vi "Qudi_HiM_QPD_PID.vi"(3 "N Z positions":i32) -> ()   [LabVIEW 2015]
uses:
  <vilib>/rvi/Analysis/control/PID/Typedef/niFpgaPID_PIGains.ctl
  <vilib>/Platform/TimedLoop/XDataNode/timing_clust.ctl
  <vilib>/Platform/TimedLoop/XDataNode/nitl_modes.ctl
  <vilib>/Platform/TimedLoop/XDataNode/wakeup.ctl
  <vilib>/rvi/FXPMathLib/basic elements/FxpIntAccumulator/subVIs/nifxpmath_IntAccumulator_SimConfig.ctl
  <vilib>/rvi/Emulation/niFpgaGetClockAttributes.vi
  <vilib>/rvi/Emulation/niFpgaSctlEmulationGetInTimedLoop.vi
  <vilib>/rvi/Emulation/niFpgaEmulationReportErrorSimple.vi
  <vilib>/rvi/eio/common/nirviEmuTemplateMethod_errors.vi
  <vilib>/rvi/Emulation/niFpgaProcessEmulError.vi
  <vilib>/rvi/Analysis/common/codeGenErrors/XNode/niFpgaXNodeCodeGenErrorHandle.vi
  <vilib>/rvi/Emulation/niFpgaCriticalErrorInLSC.vi
  <vilib>/rvi/FXPMathLib/basic elements/FxpIntAccumulator/simVIs/DllFxpIntAccumulator_sub.vi
  <vilib>/rvi/Analysis/control/PID/SubVIs/niFpgaPID_PIWrapper.vi
  <vilib>/eio/EIONode/EIONode.xnode
  <vilib>/rvi/Analysis/measure/dc-rms/XNode/niFpgaDC-RMS.xnode
  <vilib>/Platform/TimedLoop/XDataNode/XDataNode.xnode
  <vilib>/rvi/FXPMathLib/basic elements/FxpIntAccumulator/XNode/nifxpmath_IntAccumulator.xnode
  <vilib>/Platform/TimedLoop/XDataNode/XDNodeRunTimeDep.lvlib
panel:
  in  "integration_time_us":u32=100 caption="Count(uSec)"
  in  "stop":bool
  out "duration_ms":u32
  out "X":i16
  out "Y":i16
  out "Sum":i16
  out "counter":u32
  out "output":i16
  in  "reset":bool
  in  "reset_counter":bool
  in  "autofocus":bool
  in  "setpoint":i16
  in  "P":i16
  in  "I":i16
  in  "ref_axis":bool
  out "n cycles":i32
  out "DIo2":i32
  out "DIo3":i32
  out "DIo1":i32
  out "Images acquired":i32
  in  "Laser lines":i32[](array[numeric])=[0, 0, 0, 0, 0]
  in  "Laser power":i16[](array[numeric])=[0, 0, 0, 0, 0]
  in  "N laser lines":i32
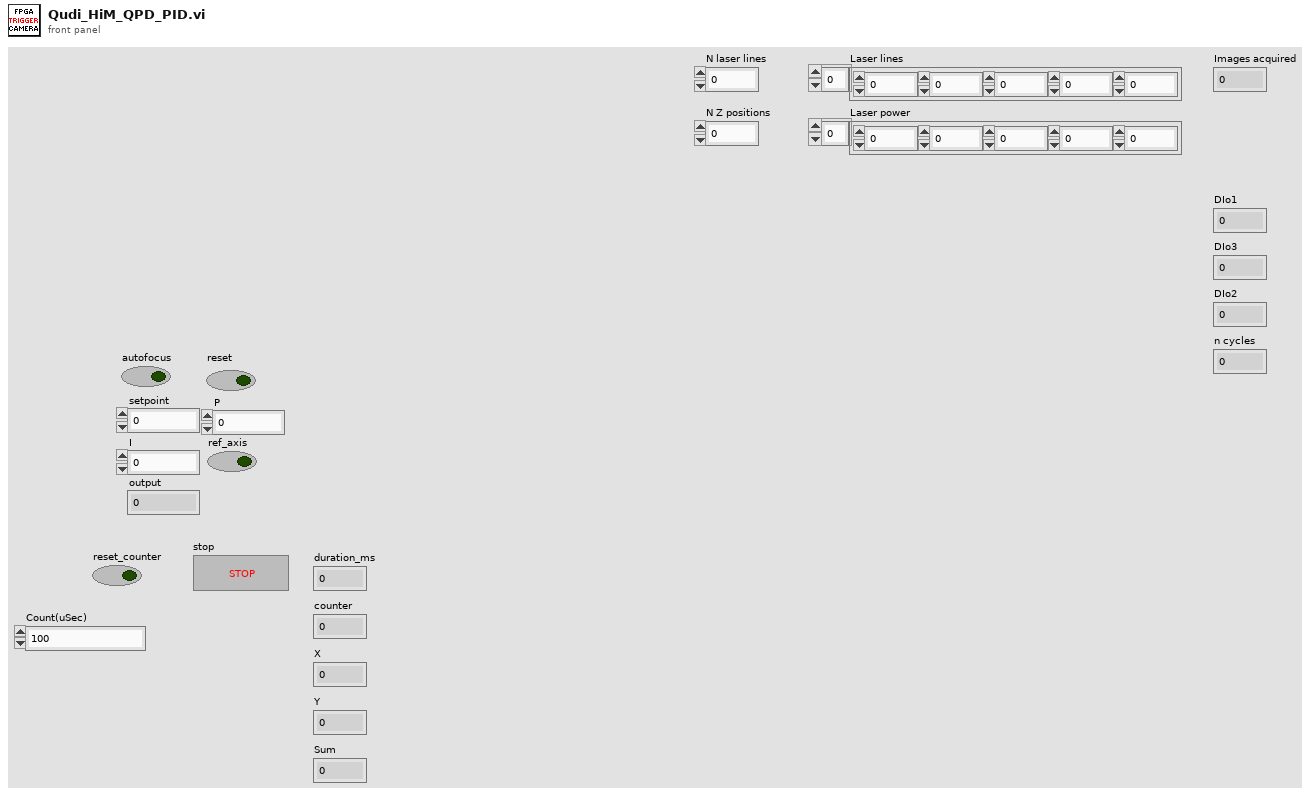
[diagram p1: front panel]
types:
  T1 = typedef "niFpgaPID_PIGains.ctl" = cluster{"proportional gain":sgl, "integral gain":sgl}
  T2 = typedef "XDNodeRunTimeDep.lvlib/timing_clust.ctl" = cluster{"Expected End [f-1]":u64, "Actual End [f-1]":u64, "Finished Late? [f-1]":bool, "Expected End [i-1]":u64, "Actual End [i-1]":u64, "Finished Late? [i-1]":bool, "Expected Start [i]":u64, "Actual Start [i]":u64, "Expected Start [f]":u64, "Actual Start [f]":u64, "Source Name":string, "Structure Name":string, "Period":i64, "Deadline":i64, "Offset":i64, "Start":i64, "Priority":i32, "Timeout":i32, "Mode":T3, "Wakeup Reason":T4, "Error":errorcluster, "Source Type":string, "Secondary Source Type":string, "Global End Time":u64, "Global Start Time":u64, "Frame Duration":u64, "Iteration Duration":u64, "Assigned CPU":i32, "I/O Scan Engine Mode":u32}
  T3 = typedef "XDNodeRunTimeDep.lvlib/nitl_modes.ctl" = enum32{"No Change", "Process missed periods, maintain original phase", "Discard missed periods, maintain original phase", "Process missed periods, ignore original phase", "Discard missed periods, ignore original phase"}
  T4 = typedef "XDNodeRunTimeDep.lvlib/wakeup.ctl" = enum32{"Normal", "Aborted", "Asynchronous wakeup", "Timing source error", "Timed loop error", "Timeout"}
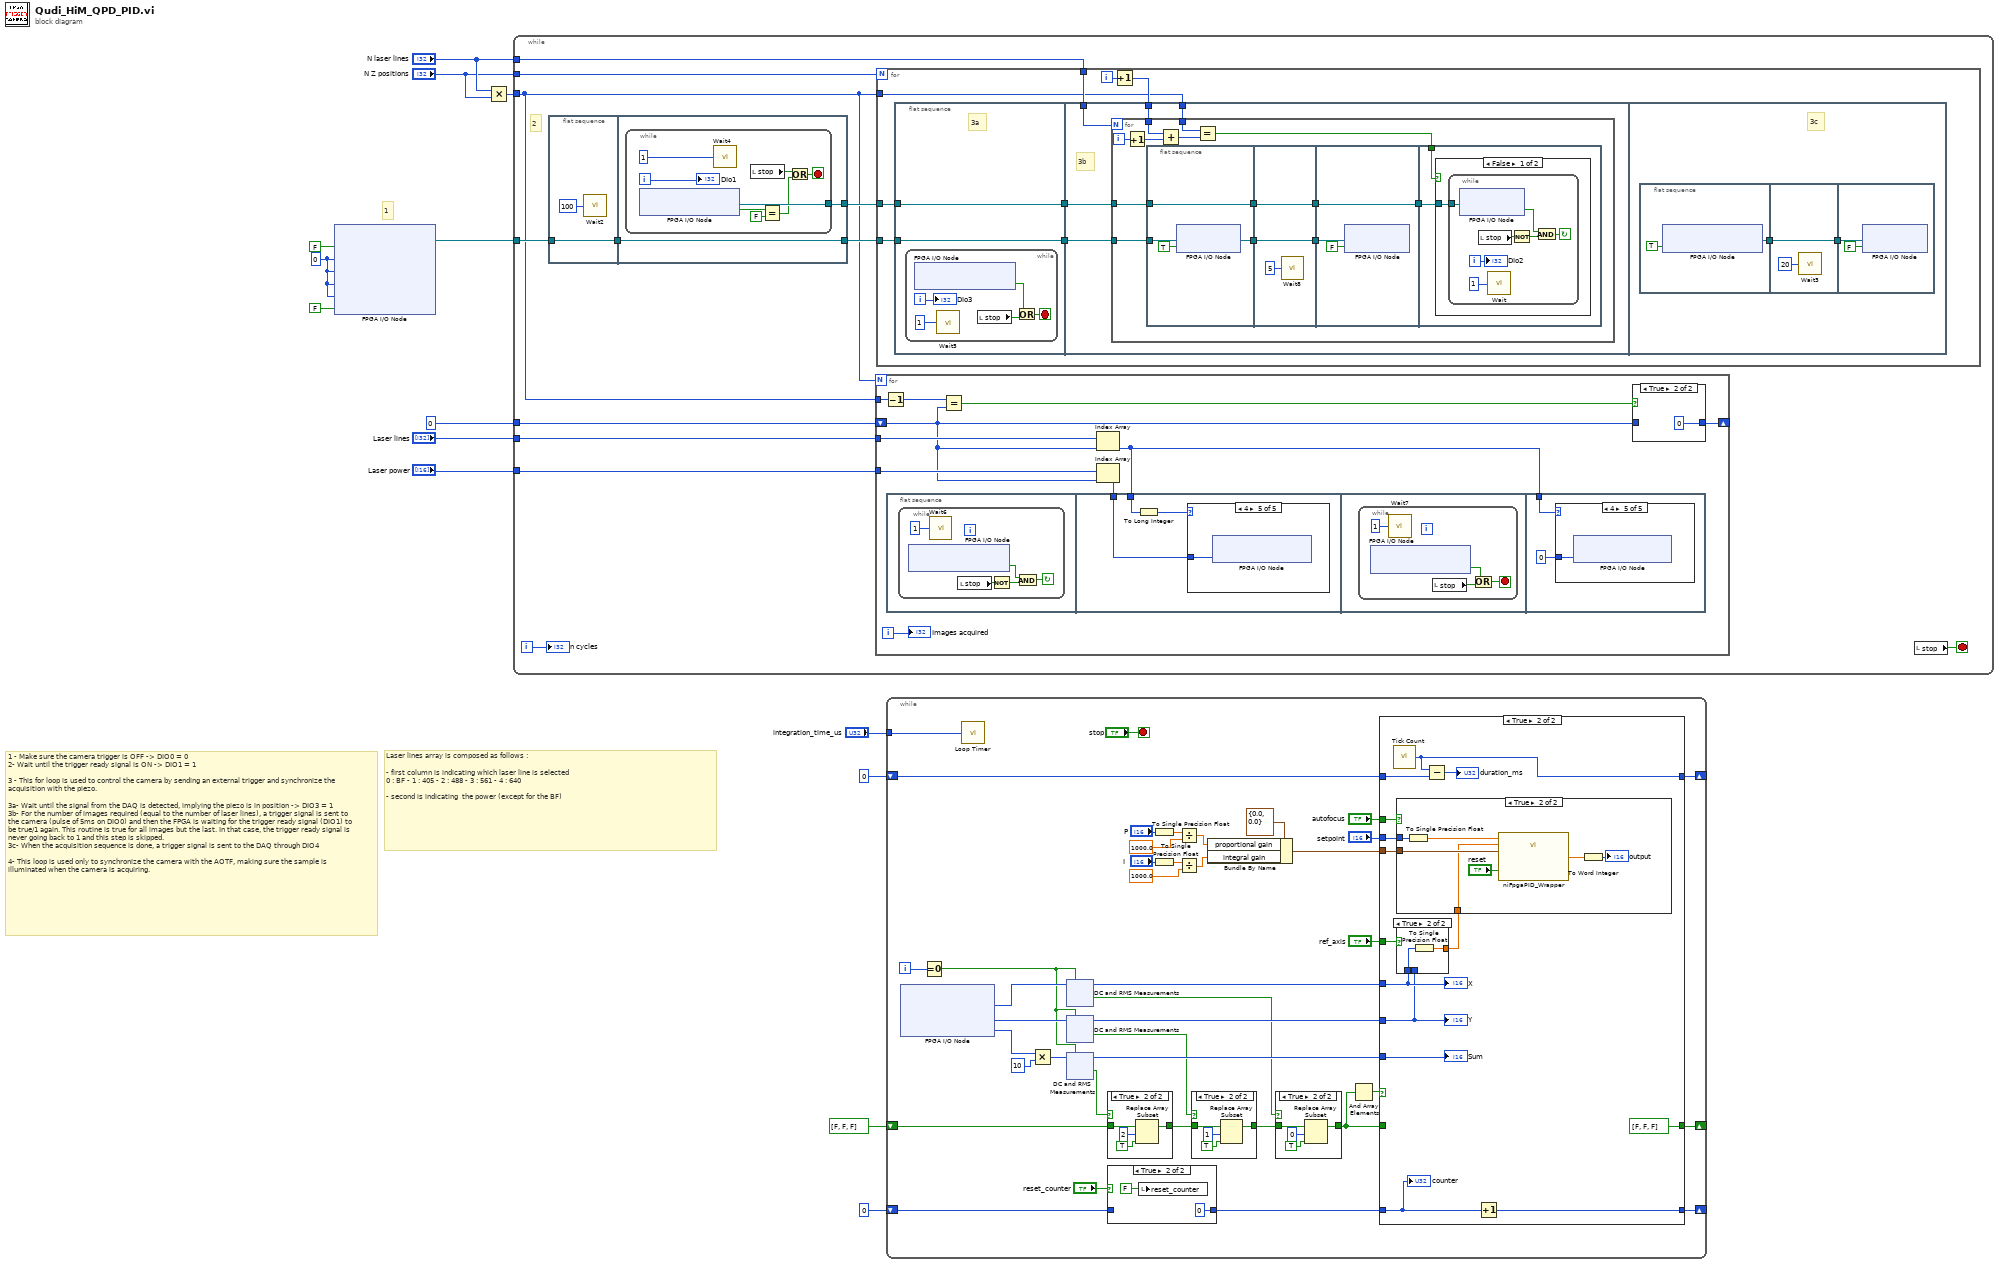
[diagram p0: block diagram]
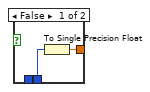
[diagram p7: hidden frame]
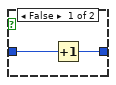
[diagram p9: hidden frame]
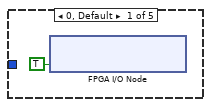
[diagram p10: hidden frame]
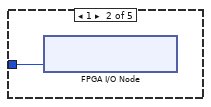
[diagram p11: hidden frame]
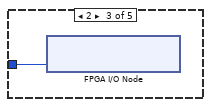
[diagram p12: hidden frame]
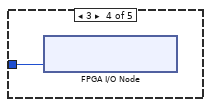
[diagram p13: hidden frame]
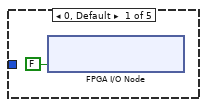
[diagram p14: hidden frame]
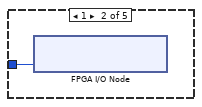
[diagram p15: hidden frame]
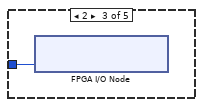
[diagram p16: hidden frame]
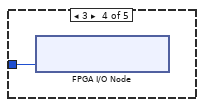
[diagram p17: hidden frame]
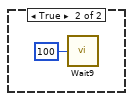
[diagram p18: hidden frame]
diagram:
  w9 = i16 0 ("Connector0/AO0")
  # "Laser lines array is composed as follows :\n\n- first column is indicating which laser line is selected \n0 : BF - 1 : 405 - 2 : 488 - 3 : 561 - 4 : 640\n\n- second is indicating  the power (except for the BF)"
  # "1"
  # "1 - Make sure the camera trigger is OFF -> DIO0 = 0\n2- Wait until the trigger ready signal is ON -> DIO1 = 1\n\n3 - This for loop is used to control the camera by sending an external trigger and synchronize the acquisition with the piezo.\n\n3a- Wait until the signal from the DAQ is detected, implying the piezo is in position -> DIO3 = 1 \n3b- For the number of images required (equal to the number of laser lines), a trigger signal is sent to the camera (pulse of 5ms on DIO0) and then the FPGA is waiting for the trigger ready signal (DIO1) to be true/1 again. This routine is true for all images but the last. In that case, the trigger ready signal is never going back to 1 and this step is skipped. \n3c- When the acquisition sequence is done, a trigger signal is sent to the DAQ through DIO4\n\n4- This loop is used only to synchronize the camera with the AOTF, making sure the sample is illuminated when the camera is acquiring."
  n1 = xnode "FPGA I/O Node"("Connector0/DIO0"=FALSE, "Connector0/AO0"=w9, "Connector0/AO1"=w9, "Connector0/AO2"=w9, "Connector0/AO3"=w9, "Connector0/DIO5"=FALSE) -> ("FPGA I/O Out"=w13:refnum<k21>)  [unwired: 6 in, 5 out]
  n2 = Multiply(x="N laser lines", y="N Z positions") -> (x*y=w1:i32)
  n3 = while {
    tunnel: w13 -> [w25]
    tunnel: "Laser power" -> [w22]
    tunnel: "Laser lines" -> [w21]
    tunnel: 0 -> [w20]
    tunnel: "N Z positions" -> [w19]
    tunnel: "N laser lines" -> [w16]
    tunnel: w1 -> [w15]
    i -> [w17]
    stop <- w18 stop-if-true
    # "2"
    n4 = flat-sequence {
      tunnel: w25 -> [w65]
      tunnel: [w65] -> w26
      tunnel: w26 -> [w67]
      tunnel: [w67] -> w24
      tunnel: [w66] -> w23
      frame #0 {
        n5 = call "Wait2"("Count(uSec)"=u32 100 ("Count(mSec)")) -> ()  [unwired: 1 out]
      }
      frame #1 {
        n6 = while {
          tunnel: [w75] -> w66
          i -> [w72]
          stop <- w68 stop-if-true
          n7 = xnode "FPGA I/O Node"() -> ("Connector0/DIO1"=w74:bool, "FPGA I/O Out"=w75:refnum<k21>)  [unwired: 1 in]
          n8 = call "Wait4"("Count(mSec)"=u32 1) -> ()  [unwired: 1 out]
          n9 = local read "stop"() -> (w69:bool)
          n10 = Equal?(x=w74, y=FALSE) -> (x = y?=w70:bool)
          n11 = Or(x=w69, y=w70) -> (x .or. y?=w68:bool)
          "DIo1" <- w72
        }
      }
    }
    n12 = for {
      N: w15 -> [_]
      shift-right: [w34] -> _
      shift-left: w20 -> [w31]
      tunnel: w21 -> [w33]
      tunnel: w22 -> [w32]
      tunnel: w15 -> [w29]
      i -> [w27]
      n13 = Decrement(x=w29) -> (x-1=w28:i32)
      n14 = flat-sequence {
        tunnel: w36 -> [w46]
        tunnel: w30 -> [w45]
        tunnel: w36 -> [w57]
        frame #0 {
          n15 = while {
            stop <- w40 continue-if-true
            n16 = xnode "FPGA I/O Node"() -> ("Connector0/DIO2"=w41:bool)  [unwired: 1 in, 1 out]
            n17 = call "Wait6"("Count(mSec)"=u32 1) -> ()  [unwired: 1 out]
            n18 = local read "stop"() -> (w42:bool)
            n19 = Not(x=w42) -> (.not. x?=w43:bool)
            n20 = And(x=w41, y=w43) -> (x .and. y?=w40:bool)
          }
        }
        frame #1 {
          n21 = To Long Integer(number=w46) -> (32bit integer=w47:i32)
          n22 = case shown="4" w47 {
            tunnel: w45 -> [_ w49 w50 w51 w52]
            frame 0, Default {
              n23 = xnode "FPGA I/O Node"("Connector0/DIO5"=TRUE) -> ()  [unwired: 1 in, 1 out]
            }
            frame 1 {
              n24 = xnode "FPGA I/O Node"("Connector0/AO2"=w49) -> ()  [unwired: 1 in, 1 out]
            }
            frame 2 {
              n25 = xnode "FPGA I/O Node"("Connector0/AO3"=w50) -> ()  [unwired: 1 in, 1 out]
            }
            frame 3 {
              n26 = xnode "FPGA I/O Node"("Connector0/AO0"=w51) -> ()  [unwired: 1 in, 1 out]
            }
            frame 4 {
              n27 = xnode "FPGA I/O Node"("Connector0/AO1"=w52) -> ()  [unwired: 1 in, 1 out]
            }
          }
        }
        frame #2 {
          n28 = while {
            stop <- w53 stop-if-true
            n29 = xnode "FPGA I/O Node"() -> ("Connector0/DIO2"=w54:bool)  [unwired: 1 in, 1 out]
            n30 = call "Wait7"("Count(mSec)"=u32 1) -> ()  [unwired: 1 out]
            n31 = local read "stop"() -> (w55:bool)
            n32 = Or(x=w54, y=w55) -> (x .or. y?=w53:bool)
          }
        }
        frame #3 {
          n33 = case shown="4" w57 {
            tunnel: i16 0 -> [_ w60 w61 w62 w63]
            frame 0, Default {
              n34 = xnode "FPGA I/O Node"("Connector0/DIO5"=FALSE) -> ()  [unwired: 1 in, 1 out]
            }
            frame 1 {
              n35 = xnode "FPGA I/O Node"("Connector0/AO2"=w60) -> ()  [unwired: 1 in, 1 out]
            }
            frame 2 {
              n36 = xnode "FPGA I/O Node"("Connector0/AO3"=w61) -> ()  [unwired: 1 in, 1 out]
            }
            frame 3 {
              n37 = xnode "FPGA I/O Node"("Connector0/AO0"=w62) -> ()  [unwired: 1 in, 1 out]
            }
            frame 4 {
              n38 = xnode "FPGA I/O Node"("Connector0/AO1"=w63) -> ()  [unwired: 1 in, 1 out]
            }
          }
        }
      }
      n39 = Equal?(x=w28, y=w31) -> (x = y?=w35:bool)
      n40 = Index Array(array=w33, index=w31) -> (element=w36:i32)
      n41 = Index Array(array=w32, index=w31) -> (element=w30:i16)
      n42 = case shown="True" w35 {
        tunnel: w31 -> [w38 _]
        tunnel: [w37 0] -> w34
        frame False {
          n43 = Increment(x=w38) -> (x+1=w37:i32)
        }
        frame True {
        }
      }
      "Images acquired" <- w27
    }
    n44 = for {
      N: w19 -> [_]
      tunnel: w24 -> [w82]
      tunnel: w23 -> [w83]
      tunnel: w16 -> [w78]
      tunnel: w15 -> [w76]
      i -> [w79]
      n45 = flat-sequence {
        tunnel: w82 -> [w84]
        tunnel: w83 -> [w85]
        tunnel: [w85] -> w81
        tunnel: [w84] -> w80
        tunnel: w81 -> [w95]
        tunnel: w80 -> [w94]
        tunnel: w78 -> [w93]
        tunnel: w77 -> [w92]
        tunnel: w76 -> [w91]
        frame #0 {
          # "3a"
          n46 = while {
            i -> [w90]
            stop <- w86 stop-if-true
            n47 = xnode "FPGA I/O Node"() -> ("Connector0/DIO3"=w87:bool)  [unwired: 1 in, 1 out]
            n48 = call "Wait5"("Count(mSec)"=u32 1) -> ()  [unwired: 1 out]
            n49 = local read "stop"() -> (w88:bool)
            n50 = Or(x=w87, y=w88) -> (x .or. y?=w86:bool)
            "DIo3" <- w90
          }
        }
        frame #1 {
          # "3b"
          n51 = for {
            N: w93 -> [_]
            tunnel: w95 -> [w103]
            tunnel: w94 -> [w102]
            tunnel: w92 -> [w99]
            tunnel: w91 -> [w97]
            i -> [w101]
            n52 = Increment(x=w101) -> (x+1=w100:i32)
            n53 = flat-sequence {
              tunnel: [w111] -> w108
              tunnel: [w109] -> w107
              tunnel: w102 -> [w110]
              tunnel: w103 -> [w109]
              tunnel: w108 -> [w115]
              tunnel: [w115] -> w106
              tunnel: [w114] -> w105
              tunnel: w107 -> [w114]
              tunnel: w106 -> [w117]
              tunnel: [w116] -> w104
              tunnel: w105 -> [w116]
              tunnel: w104 -> [w120]
              tunnel: w96 -> [w119]
              frame #0 {
                n54 = xnode "FPGA I/O Node"("I/O Item"=TRUE ("Connector0/DIO0"), "FPGA I/O In"=w110) -> ("FPGA I/O Out"=w111:refnum<k21>)
              }
              frame #1 {
                n55 = call "Wait8"("Count(mSec)"=u32 5) -> ()  [unwired: 1 out]
              }
              frame #2 {
                n56 = xnode "FPGA I/O Node"("I/O Item"=FALSE ("Connector0/DIO0"), "FPGA I/O In"=w117) -> ()  [unwired: 1 out]
              }
              frame #3 {
                n57 = case shown="False" w119 {
                  tunnel: w120 -> [w121 _]
                  frame False {
                    n58 = while {
                      tunnel: w121 -> [w128]
                      i -> [w127]
                      stop <- w122 continue-if-true
                      n59 = xnode "FPGA I/O Node"("FPGA I/O In"=w128) -> ("I/O Item"=w123:bool)  [unwired: 1 out]
                      n60 = local read "stop"() -> (w125:bool)
                      n61 = call "Wait"("Count(mSec)"=u32 1) -> ()  [unwired: 1 out]
                      n62 = Not(x=w125) -> (.not. x?=w124:bool)
                      n63 = And(x=w123, y=w124) -> (x .and. y?=w122:bool)
                      "DIo2" <- w127
                    }
                  }
                  frame True {
                    n64 = call "Wait9"("Count(uSec)"=u32 100 ("Count(mSec)")) -> ()  [unwired: 1 out]
                  }
                }
              }
            }
            n65 = Add(x=w99, y=w100) -> (x+y=w98:i32)
            n66 = Equal?(x=w97, y=w98) -> (x = y?=w96:bool)
          }
        }
        frame #2 {
          # "3c"
          n67 = flat-sequence {
            tunnel: [w133] -> w131
            tunnel: w131 -> [w134]
            tunnel: [w134] -> w130
            tunnel: w130 -> [w136]
            frame #0 {
              n68 = xnode "FPGA I/O Node"("Connector0/DIO4"=TRUE) -> ("FPGA I/O Out"=w133:refnum<k21>)  [unwired: 1 in]
            }
            frame #1 {
              n69 = call "Wait3"("Count(mSec)"=u32 20) -> ()  [unwired: 1 out]
            }
            frame #2 {
              n70 = xnode "FPGA I/O Node"("I/O Item"=FALSE ("Connector0/DIO0"), "FPGA I/O In"=w136) -> ()  [unwired: 1 out]
            }
          }
        }
      }
      n71 = Increment(x=w79) -> (x+1=w77:i32)
    }
    n72 = local read "stop"() -> (w18:bool)
    "n cycles" <- w17
  }
  n73 = while {
    shift-right: [w161] -> _
    shift-left: bool[] [FALSE, FALSE, FALSE] ("initialized array") -> [w169]
    shift-right: [w159] -> _
    shift-left: u32 0 -> [w160]
    tunnel: "integration_time_us" -> [w158]
    shift-right: [w157] -> _
    shift-left: u32 0 -> [w155]
    i -> [w175]
    stop <- "stop" stop-if-true
    n74 = xnode "FPGA I/O Node"() -> ("Connector0/AI0"=w177:i16, "Connector0/AI1"=w173:i16, "Connector0/AI2"=w140:i16)  [unwired: 3 in, 3 out]
    n75 = Equal To 0?(x=w175) -> (x = 0?=w170:bool)
    n76 = call "Loop Timer"("Count(uSec)"=w158) -> ()  [unwired: 1 out]
    n77 = Multiply(x=w140, y=i16 10) -> (x*y=w139:i16)
    n78 = xnode "DC and RMS Measurements"("input data"=w177, "reset"=w170) -> ("DC"=w174:i16, "output valid"=w164:bool)
    n79 = xnode "DC and RMS Measurements"("input data"=w173, "reset"=w170) -> ("DC"=w172:i16, "output valid"=w165:bool)
    n80 = xnode "DC and RMS Measurements"("input data"=w139, "reset"=w170) -> ("DC"=w171:i16, "output valid"=w166:bool)
    n81 = case shown="True" w166 {
      tunnel: w169 -> [w186 w189]
      tunnel: [w186 w187] -> w168
      frame False {
      }
      frame True {
        n82 = Replace Array Subset(array=w189, new element=TRUE, index=2) -> (w187:bool[])
      }
    }
    n83 = case shown="True" "reset_counter" {
      tunnel: w155 -> [w178 _]
      tunnel: [w178 u32 0] -> w154
      frame False {
      }
      frame True {
        n84 = local write "reset_counter"(FALSE ("Reset counter")) -> ()
      }
    }
    n85 = To Single Precision Float(number="P") -> (single precision float=w147:sgl)
    n86 = To Single Precision Float(number="I") -> (single precision float=w144:sgl)
    n87 = Divide(x=w147, y=sgl 1000.0) -> (x/y=w145:sgl)
    n88 = Divide(x=w144, y=sgl 1000.0) -> (x/y=w142:sgl)
    n89 = case shown="True" w165 {
      tunnel: w168 -> [w191 w194]
      tunnel: [w191 w192] -> w167
      frame False {
      }
      frame True {
        n90 = Replace Array Subset(array=w194, new element=TRUE, index=1) -> (w192:bool[])
      }
    }
    n91 = Bundle By Name(cluster=T1 {"proportional gain"=0.0, "integral gain"=0.0} ("gains"), "proportional gain"=w145, "integral gain"=w142) -> (w148:T1)
    n92 = case shown="True" w164 {
      tunnel: [w181 w183] -> w162
      tunnel: w167 -> [w181 w182]
      frame False {
      }
      frame True {
        n93 = Replace Array Subset(array=w182, new element=TRUE, index=0) -> (w183:bool[])
      }
    }
    n94 = And Array Elements(Boolean array=w162) -> (logical AND=w163:bool)
    n95 = case shown="True" w163 {
      tunnel: w174 -> [_ w201]
      tunnel: w172 -> [_ w199]
      tunnel: w171 -> [_ w207]
      tunnel: w162 -> [w198 _]
      tunnel: [w198 bool[] [FALSE, FALSE, FALSE] ("initialized array")] -> w161
      tunnel: w160 -> [w197 w211]
      tunnel: [w197 w209] -> w159
      tunnel: w154 -> [w196 w206]
      tunnel: [w196 w208] -> w157
      tunnel: "autofocus" -> [_ w205]
      tunnel: "setpoint" -> [_ w204]
      tunnel: w148 -> [_ w203]
      tunnel: "ref_axis" -> [_ w202]
      frame False {
      }
      frame True {
        n96 = call "Tick Count"() -> ("Tick Count(mSec)"=w209:u32)
        n97 = case shown="True" w202 {
          tunnel: w201 -> [_ w216]
          tunnel: [w213 w215] -> w200
          tunnel: w199 -> [w214 _]
          frame False {
            n98 = To Single Precision Float(number=w214) -> (single precision float=w213:sgl)
          }
          frame True {
            n99 = To Single Precision Float(number=w216) -> (single precision float=w215:sgl)
          }
        }
        n100 = case shown="True" w205 {
          tunnel: w204 -> [_ w223]
          tunnel: w203 -> [_ w221]
          tunnel: w200 -> [_ w217]
          frame False {
          }
          frame True {
            n101 = To Single Precision Float(number=w223) -> (single precision float=w222:sgl)
            n102 = call-poly <vilib>:"niFpgaPID_Wrapper.vi"("setpoint"=w222, "reset? (F)"="reset", "process variable"=w217, "gains"=w221) -> ("output"=w219:sgl)  [unwired: 9 in, 2 out]
            n103 = To Word Integer(number=w219) -> (16bit integer=→"output":i16)
          }
        }
        n104 = Subtract(x=w209, y=w211) -> (x-y=→"duration_ms":u32)
        n105 = Increment(x=w206) -> (x+1=w208:u32)
        "X" <- w201
        "Y" <- w199
        "Sum" <- w207
        "counter" <- w206
      }
    }
  }
